vi "SequenceNodeUI.vi"() -> ()   [LabVIEW 2015, in "SequenceNode.lvclass"]
doc: "Copyright 2017 National Instruments Corporation\n\nLicensed under the Apache License, Version 2.0 (the \"License\"); you may not use this file except in compliance with the License. You may obtain a copy of the License at http://www.apache.org/licenses/LICENSE-2.0\nUnless required by applicable law or agreed to in writing, software distributed under the License is distributed on an \"AS IS\" BASIS, WITHOUT WARRANTIES OR CONDITIONS OF ANY KIND, either express or implied. See the License for the specific language governing permissions and limitations under the License."
uses:
  SequenceNode.lvclass
  <vilib>/NI/Configuration Framework/Node/NodeRef.ctl
  <vilib>/NI/Configuration Framework/Node/NISE_CEF_Node.lvclass
  <vilib>/NI/AMC/Message Queue.ctl
  <vilib>/NI/AMC/Message.ctl
  <vilib>/NI/Tools/Keyed Array/KeyedArray.ctl
  <vilib>/NI/Configuration Framework/Node/UserEventRef.ctl
  <vilib>/NI/Configuration Framework/Controls/EventCluster.ctl
  <vilib>/NI/AMC/Create Single Message.vi
  <vilib>/NI/AMC/Update Message Routing Info.vi
  <vilib>/NI/AMC/Send Message.vi
  Prototype/classes/Sequence/Config/Sequence Config.lvclass
  <vilib>/NI/AMC/AMC.lvlib
  <vilib>/NI/Tools/Keyed Array/Tools_KeyedArray.lvlib
  <vilib>/NI/Configuration Framework/NISE_CEF_TreeControl.lvlib
panel:
  out "Sequence Version":string
  in  "user event":T1
  in  "main queue":T2
  in  "Sequence Name":string
  in  "node ref":T3
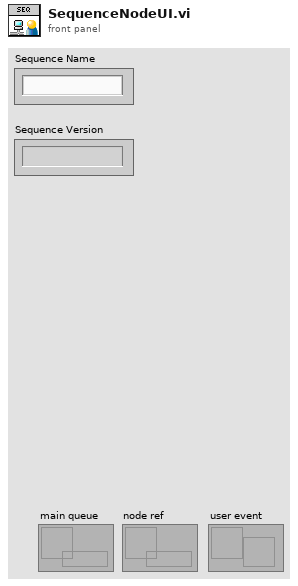
[diagram p1: front panel]
types:
  T1 = typedef "NISE_CEF_Node.lvclass/UserEventRef.ctl" = refnum<user-event>
  T2 = typedef "AMC.lvlib/Message Queue.ctl" = refnum<queue>
  T3 = typedef "NISE_CEF_Node.lvclass/NodeRef.ctl" = refnum<data-value>
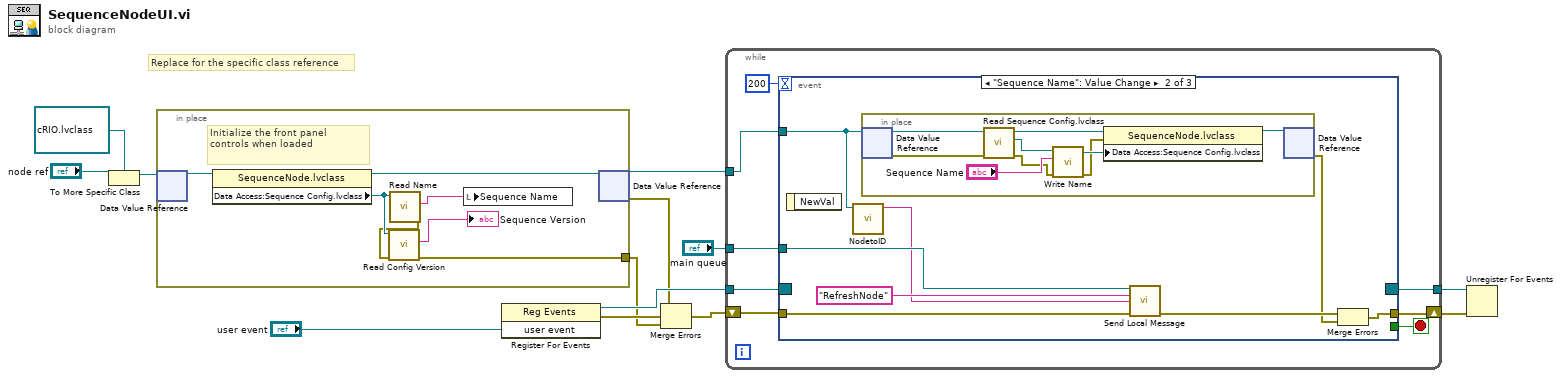
[diagram p0: block diagram]
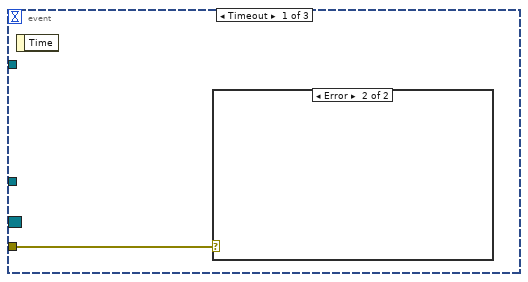
[diagram p2: hidden frame]
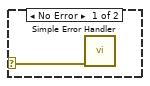
[diagram p3: hidden frame]
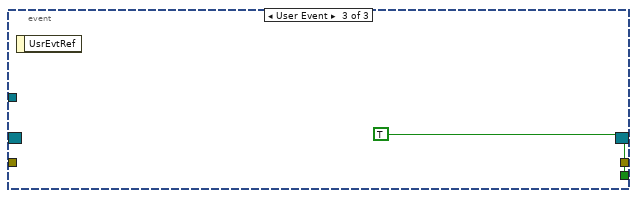
[diagram p4: hidden frame]
diagram:
  # "Replace for the specific class reference"
  n1 = To More Specific Class(target class=refnum<data-value> refnum ("data value reference"), reference="node ref") -> (specific class reference=w6:refnum<data-value>)  [unwired: 1 in, 1 out]
  n2 = in-place {
    in-place-border: [w14] -> w1
    # "Initialize the front panel controls when loaded"
    n3 = in-place-dvr #1(w6) -> (w20:refnum<class "SequenceNode.lvclass">)  [unwired: 1 out]
    n4 = property class="SequenceNode.lvclass"(reference=w20) -> (reference out=w19:refnum<class "SequenceNode.lvclass">, "Data Access:Sequence Config.lvclass"=w16:refnum<class "Sequence Config.lvclass">)  [unwired: 1 in, 1 out]
    n5 = call-dynamic "Read Name.vi"("Sequence in"=w16) -> ("error out"=w15:errorcluster, "Name"=w18:string)  [unwired: 8 in, 1 out]
    n6 = call-dynamic "Read Config Version.vi"("error in (no error)"=w15, "Sequence Config in"=w16) -> ("error out"=w14:errorcluster, "String"=→"Sequence Version":string)  [unwired: 7 in, 1 out]
    n7 = local write "Sequence Name"(w18) -> ()
    n8 = in-place-dvr #1(w19) -> (w13:refnum<data-value>, w3:errorcluster)
  }
  n9 = register-events("user event") -> (reference out=w10:refnum<event-registration>, error out=w4:errorcluster)  [unwired: 2 in]
  n10 = Merge Errors(w3, w4, w1) -> (w2:errorcluster)
  n11 = while {
    tunnel: w13 -> [w28]
    tunnel: "main queue" -> [w27]
    tunnel: w10 -> [w25]
    tunnel: [w24] -> w9
    shift-right: [w22] -> w8
    shift-left: w2 -> [w21]
    stop <- w23 stop-if-true
    n12 = event shown="[1] \"Sequence Name\": Value Change" {
      selector: w25 -> [_ _ _]
      dyn-events: [_ _ _] -> w24
      timeout: 200 -> [_ _ _]
      tunnel: w28 -> [_ w36 _]
      tunnel: w27 -> [_ w37 _]
      tunnel: [_ _ TRUE] -> w23
      tunnel: [_ w32 _] -> w22
      tunnel: w21 -> [w29 w33 _]
      event Timeout {
        n13 = event-data() -> ()  [unwired: 1 in, 1 out]
        n14 = case shown="Error" w29 {
          selector: w29 -> [w30 _]
          frame No Error {
            n15 = call <vilib>:"Simple Error Handler.vi"("error in (no error)"=w30) -> ()  [unwired: 4 in, 5 out]
          }
          frame Error {
          }
        }
      }
      event "Sequence Name": Value Change {
        n16 = event-data() -> ()  [unwired: 1 in, 1 out]
        n17 = call <vilib>:"NodetoID.vi"("node ref"=w36) -> ("ID"=w35:string)  [unwired: 9 in, 1 out]
        n18 = in-place {
          n19 = in-place-dvr #2(w36) -> (w47:refnum<class "SequenceNode.lvclass">, w41:errorcluster)
          n20 = call-dynamic "Read Sequence Config.lvclass.vi"("error in (no error)"=w41, "SequenceNode in"=w47) -> ("error out"=w40:errorcluster, "Sequence Config.lvclass"=w42:refnum<class "Sequence Config.lvclass">, "SequenceNode out"=w43:refnum<class "SequenceNode.lvclass">)  [unwired: 7 in]
          n21 = call-dynamic "Write Name.vi"("error in (no error)"=w40, "Name"="Sequence Name", "Sequence in"=w42) -> ("error out"=w39:errorcluster, "Sequence out"=w44:refnum<class "Sequence Config.lvclass">)  [unwired: 7 in]
          n22 = property class="SequenceNode.lvclass"(reference=w43, error in=w39, "Data Access:Sequence Config.lvclass"=w44) -> (reference out=w46:refnum<class "SequenceNode.lvclass">)  [unwired: 1 out]
          n23 = in-place-dvr #2(w46) -> (w31:errorcluster)  [unwired: 1 out]
        }
        n24 = call <vilib>:"Send Local Message.vi"("message queue in"=w37, "message name"="RefreshNode" ("Message Name"), "message value"=w35, "error in"=w33) -> ("error out"=w34:errorcluster)  [unwired: 9 in, 2 out]
        n25 = Merge Errors(w34, w31) -> (w32:errorcluster)
      }
      event User Event {
        n26 = event-data() -> ()  [unwired: 1 in, 1 out]
      }
    }
  }
  n27 = Unregister For Events(event registration refnum=w9, error in=w8) -> ()  [unwired: 1 out]
